vi "GetYPRfromQuaternion.vi"(11 "qa":T1) -> (1 "YPR Deg (out)":cluster{"Yaw":dbl, "Pitch":dbl, "Roll":dbl}, 3 "YPR Radiens (out)":cluster{"Yaw":dbl, "Pitch":dbl, "Roll":dbl})   [LabVIEW 2015]
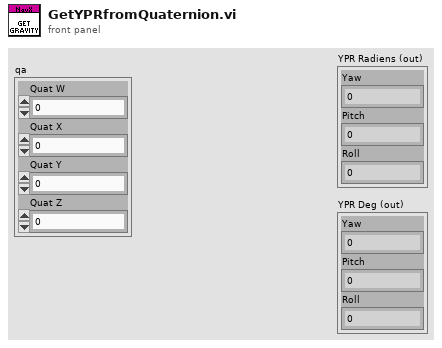
[diagram p1: front panel]
types:
  T1 = cluster{"Quat W":dbl, "Quat X":dbl, "Quat Y":dbl, "Quat Z":dbl}
  T2 = cluster{"Gravity X":dbl, "Gravity Y":dbl, "Gravity Z":dbl}
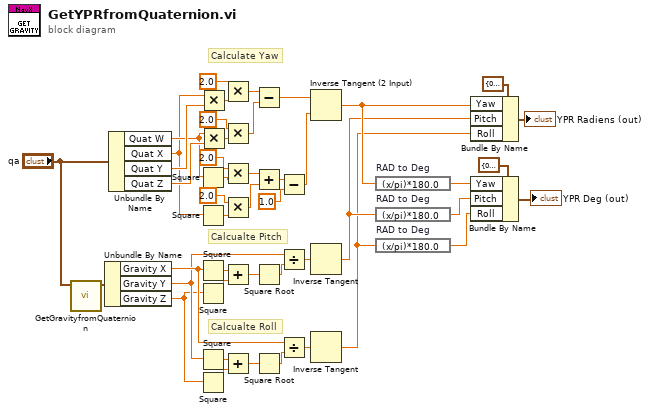
[diagram p0: block diagram]
diagram:
  # "Calcualte Roll"
  # "Calculate Yaw"
  # "Calcualte Pitch"
  n1 = call "GetGravityfromQuaternion.vi"("qa"="qa") -> ("Gravity (out)"=w42:T2)  [unwired: 10 in]
  n2 = Unbundle By Name(w42) -> ("Gravity X"=w36:dbl, "Gravity Y"=w30:dbl, "Gravity Z"=w29:dbl)
  n3 = Unbundle By Name("qa") -> ("Quat W"=w16:dbl, "Quat X"=w15:dbl, "Quat Y"=w18:dbl, "Quat Z"=w17:dbl)
  n4 = Square(x=w16) -> (x^2=w13:dbl)
  n5 = Square(x=w15) -> (x^2=w10:dbl)
  n6 = Square(x=w36) -> (x^2=w41:dbl)
  n7 = Square(x=w29) -> (x^2=w40:dbl)
  n8 = Square(x=w30) -> (x^2=w33:dbl)
  n9 = Square(x=w29) -> (x^2=w34:dbl)
  n10 = Multiply(x=w15, y=w18) -> (x*y=w27:dbl)
  n11 = Multiply(x=w16, y=w17) -> (x*y=w25:dbl)
  n12 = Multiply(x=2.0, y=w27) -> (x*y=w26:dbl)
  n13 = Multiply(x=2.0, y=w25) -> (x*y=w23:dbl)
  n14 = Multiply(x=2.0, y=w13) -> (x*y=w12:dbl)
  n15 = Multiply(x=2.0, y=w10) -> (x*y=w9:dbl)
  n16 = Add(x=w41, y=w40) -> (x+y=w39:dbl)
  n17 = Add(x=w33, y=w34) -> (x+y=w35:dbl)
  n18 = Subtract(x=w26, y=w23) -> (x-y=w20:dbl)
  n19 = Add(x=w12, y=w9) -> (x+y=w22:dbl)
  n20 = Square Root(x=w39) -> (sqrt(x)=w38:dbl)
  n21 = Square Root(x=w35) -> (sqrt(x)=w32:dbl)
  n22 = Subtract(x=w22, y=1.0 ("x")) -> (x-y=w19:dbl)
  n23 = Divide(x=w30, y=w38) -> (x/y=w37:dbl)
  n24 = Divide(x=w36, y=w32) -> (x/y=w31:dbl)
  n25 = Inverse Tangent (2 Input)(1:w19, 2:w20) -> (0:w8:dbl)
  n26 = Inverse Tangent(1:w37) -> (0:w5:dbl)
  n27 = Inverse Tangent(1:w31) -> (0:w4:dbl)
  n28 = expression code="(x/pi)*180.0" "RAD to Deg"(w8) -> (w1:dbl)
  n29 = expression code="(x/pi)*180.0" "RAD to Deg"(w5) -> (w2:dbl)
  n30 = expression code="(x/pi)*180.0" "RAD to Deg"(w4) -> (w3:dbl)
  n31 = Bundle By Name(cluster=cluster{"Yaw":dbl, "Pitch":dbl, "Roll":dbl} {"Yaw"=0.0, "Pitch"=0.0, "Roll"=0.0} ("YPR (out)"), "Yaw"=w8, "Pitch"=w5, "Roll"=w4) -> (→"YPR Radiens (out)":cluster{"Yaw":dbl, "Pitch":dbl, "Roll":dbl})
  n32 = Bundle By Name(cluster=cluster{"Yaw":dbl, "Pitch":dbl, "Roll":dbl} {"Yaw"=0.0, "Pitch"=0.0, "Roll"=0.0} ("YPR (out)"), "Yaw"=w1, "Pitch"=w2, "Roll"=w3) -> (→"YPR Deg (out)":cluster{"Yaw":dbl, "Pitch":dbl, "Roll":dbl})
